vi "DialogCloneClass.vi"(0 "ClassWriterNative.lvclass":refnum<class "ClassWriterNative.lvclass">, 1 "ClassItemRefIn":refnum<vi>, 5 "error in (no error)":errorcluster) -> (14 "ClassWriterGOOP300.lvclassOut":refnum<class "ClassWriterNative.lvclass">, 15 "ClassItemRefOut":refnum<vi>, 16 "NewClassPath":path, 17 "Cancelled":bool, 19 "error out":errorcluster)   [LabVIEW 2014, in "ClassWriterNative.lvclass"]
uses:
  <resource>/Framework/Providers/Open_GDS/ClassProviders/Provider_LvNativeClass/ClassWriterNative_class/ClassWriterNative.lvclass
  <resource>/Framework/Providers/Open_GDS/SubVIs/GOOP_HelpButton.ctl
  <vilib>/Utility/lvfile.llb/NI_FileType.lvlib
panel:
  out "ProductPicture":picture
  in  "_HelpCloneClass":T1
  in  "_UseClassSuffix":string caption="Class Folder Suffix"
  in  "_NewClassPath":path caption="New Class Folder"
  in  "_NewClassName":string caption="New Class Name"
  out "_DubName":string caption="This class already exists"
  in  "_Cancel":bool
  in  "_CloneClass":bool
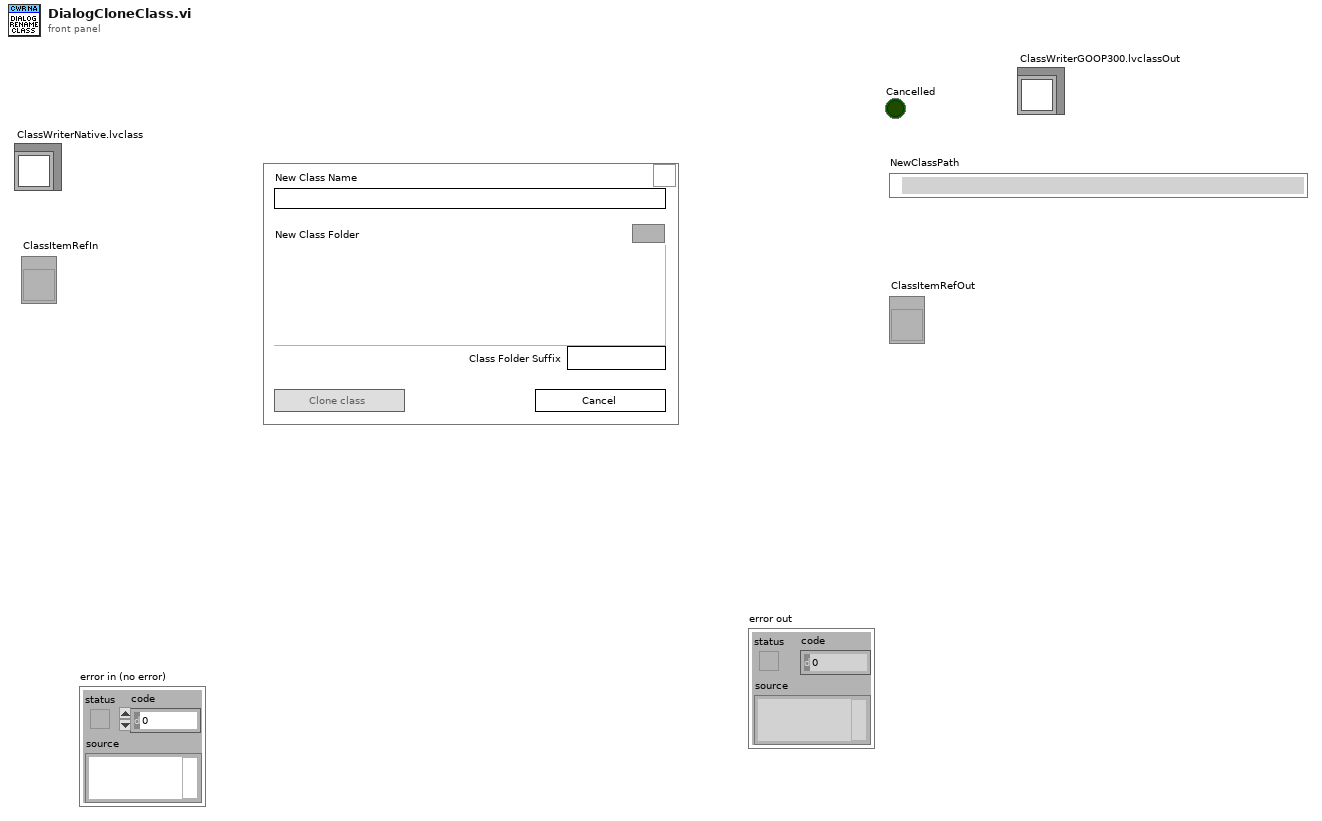
[diagram p1: front panel]
types:
  T1 = typedef "GOOP_HelpButton.ctl" = bool
  T2 = cluster{"Cancel":bool, "OrgClassPath":path, "ClassName":string}
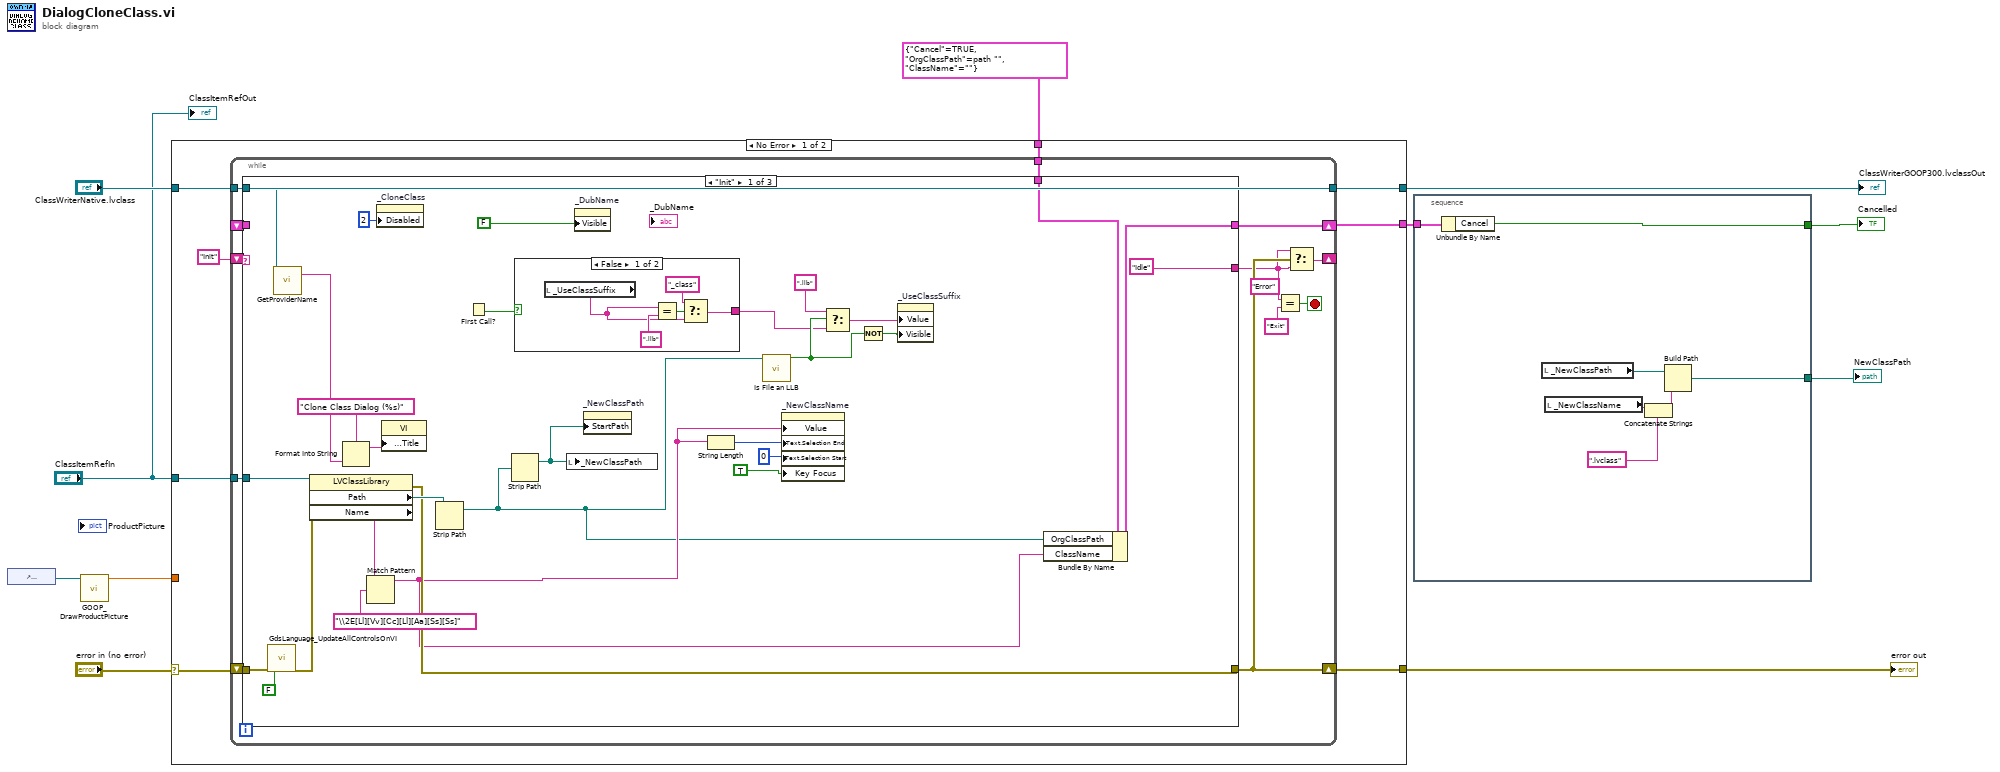
[diagram p0: block diagram]
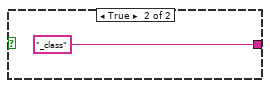
[diagram p2: hidden frame]
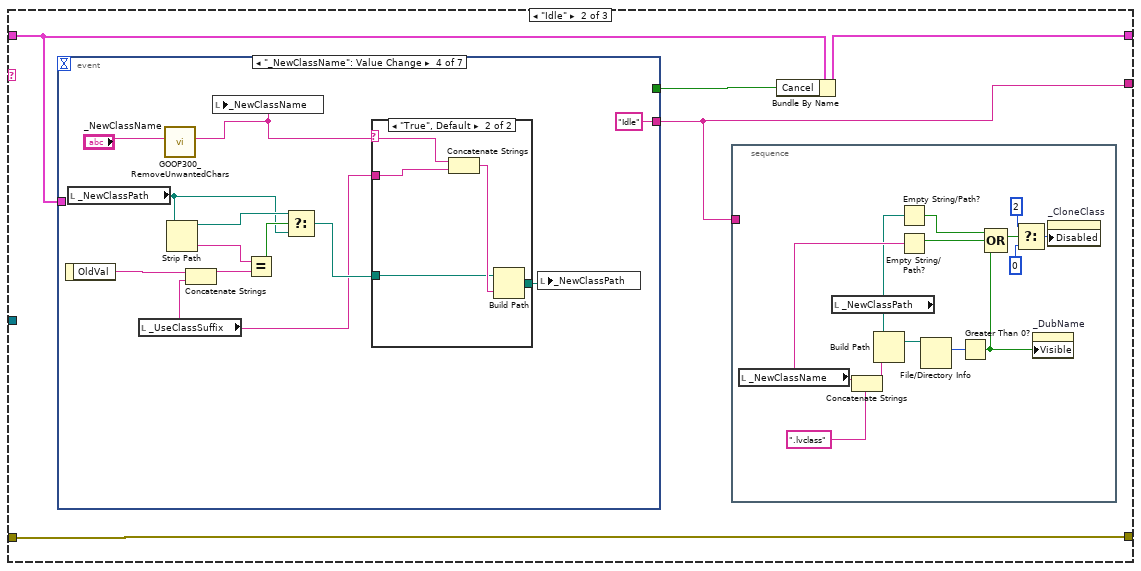
[diagram p3: hidden frame]
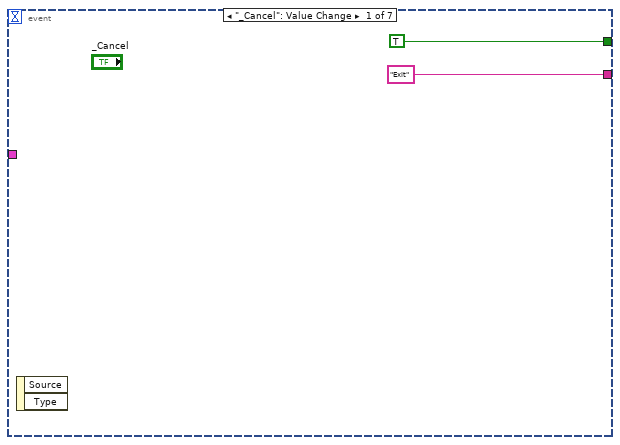
[diagram p4: hidden frame]
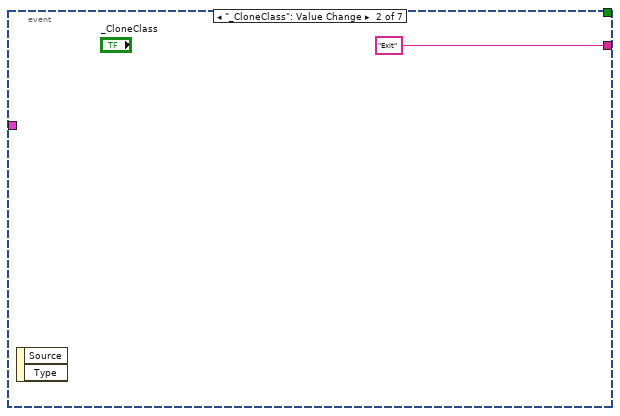
[diagram p5: hidden frame]
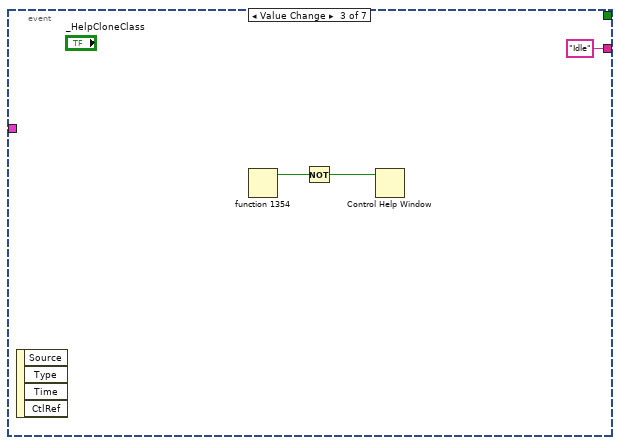
[diagram p6: hidden frame]
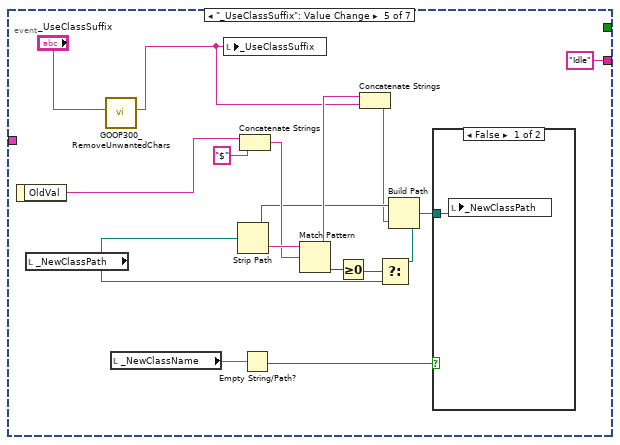
[diagram p8: hidden frame]
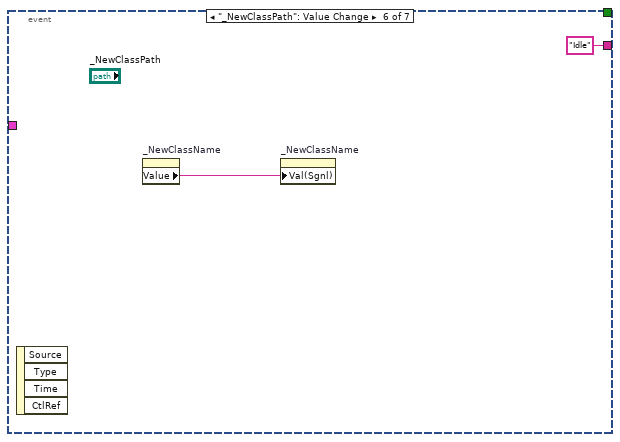
[diagram p10: hidden frame]
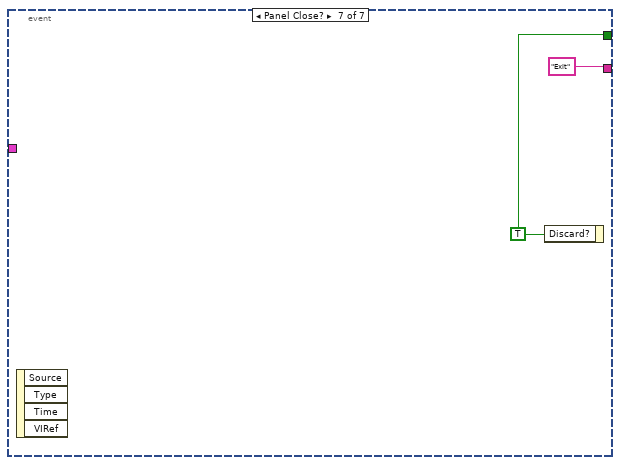
[diagram p11: hidden frame]
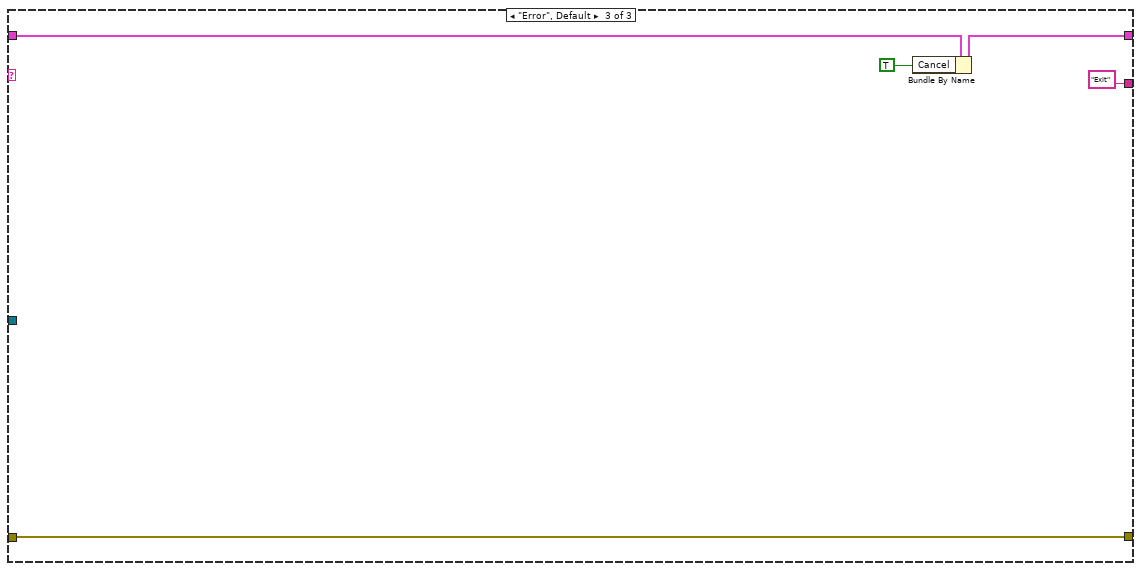
[diagram p12: hidden frame]
diagram:
  n1 = control-ref of="ProductPicture"() -> (w2:refnum<vi>)
  n2 = call <resource>:"GOOP_DrawProductPicture.vi"("ProductPictureControl"=w2) -> ("Zoom Factor"=w1:sgl)  [unwired: 10 in]
  n3 = case shown="No Error" "error in (no error)" {
    selector: "error in (no error)" -> [w19 w137]
    tunnel: "ClassWriterNative.lvclass" -> [w15 w136]
    tunnel: [w18 w137] -> w5
    tunnel: [w16 w136] -> w9
    tunnel: T2 {"Cancel"=TRUE, "OrgClassPath"=path "", "ClassName"=""} ("output cluster") -> [w14 _]
    tunnel: "ClassItemRefIn" -> [w13 _]
    tunnel: [w12 _] -> w8
    tunnel: w1 -> [_ _]
    frame No Error {
      n4 = while {
        shift-right: [w26] -> w18
        shift-left: w19 -> [w32]
        shift-right: [w25] -> _
        shift-left: "Init" -> [w29]
        shift-right: [w30] -> w12
        shift-left: _ -> [w31]
        tunnel: w15 -> [w22]
        tunnel: [w22] -> w16
        tunnel: w14 -> [w21]
        tunnel: w13 -> [w20]
        stop <- w27 stop-if-true
        n5 = case shown="\"Init\"" w29 {
          tunnel: w31 -> [_ w68 w133]
          tunnel: [w60 w70 w132] -> w30
          tunnel: w32 -> [w41 w72 w134]
          tunnel: [w52 w72 w134] -> w26
          tunnel: w22 -> [w43 _ _]
          tunnel: ["Idle" w71 "Exit"] -> w24
          tunnel: w21 -> [w58 _ _]
          tunnel: w20 -> [w59 _ _]
          frame "Init" {
            n6 = call <resource>:"GdsLanguage_UpdateAllControlsOnVI.vi"("error in (no error)"=w41, "CreateLanguageFile(Use this to create a languageFile)"=FALSE) -> ("error out"=w40:errorcluster)  [unwired: 16 in, 1 out]
            n7 = call-dynamic "GetProviderName.vi"("ClassWriterNative in"=w43) -> ("ProviderName"=w42:string)  [unwired: 16 in, 2 out]
            n8 = property class="LVClassLibrary"(reference=w59, error in=w40) -> (error out=w52:errorcluster, "Path"=w56:path, "Name"=w55:string)  [unwired: 1 out]
            n9 = Format Into String(format string="Clone Class Dialog (%s)", w42) -> (resulting string=w45:string)  [unwired: 2 in, 1 out]
            n10 = Match Pattern(string=w55, regular expression="\\2E[Ll][Vv][Cc][Ll][Aa][Ss][Ss]") -> (before substring=w50:string)  [unwired: 1 in, 3 out]
            n11 = property on="_CloneClass" class="Bool"("Disabled"=u8 2) -> ()  [unwired: 2 in, 2 out]
            n12 = property class="VI"("Front Panel.Title"=w45) -> ()  [unwired: 2 in, 2 out]
            n13 = Strip Path(path=w56) -> (stripped path=w33:path)  [unwired: 1 out]
            n14 = First Call?() -> (First Call?: T/F=w48:bool)
            n15 = Strip Path(path=w33) -> (stripped path=w47:path)  [unwired: 1 out]
            n16 = case shown="False" w48 {
              tunnel: [w63 "_class" ("Use Class Prefix")] -> w34
              frame False {
                n17 = local read "_UseClassSuffix"() -> (w62:string)
                n18 = Equal?(x=w62, y=".llb") -> (x = y?=w66:bool)
                n19 = Select(t="_class" ("Use Class Prefix"), s=w66, f=w62) -> (s? t:f=w63:string)
              }
              frame True {
              }
            }
            n20 = local write "_NewClassPath"(w47) -> ()
            n21 = property on="_DubName" class="Str"("Visible"=FALSE) -> ()  [unwired: 2 in, 2 out]
            n22 = property on="_NewClassPath" class="Path"("StartPath"=w47) -> ()  [unwired: 2 in, 2 out]
            n23 = String Length(string=w50) -> (length=w46:i32)
            n24 = call <vilib>:"Is File an LLB.vi"("path"=w33) -> ("Is LLB?"=w35:bool)  [unwired: 9 in, 1 out]
            n25 = property on="_NewClassName" class="Str"("Value"=w50, "Text.Selection End"=w46, "Text.Selection Start"=u32 0 ("Text.Selection:Start"), "Key Focus"=TRUE) -> ()  [unwired: 2 in, 2 out]
            n26 = Select(t=".llb" ("y"), s=w35, f=w34) -> (s? t:f=w36:string)
            n27 = Not(x=w35) -> (.not. x?=w38:bool)
            n28 = property on="_UseClassSuffix" class="Str"("Value"=w36, "Visible"=w38) -> ()  [unwired: 2 in, 2 out]
            n29 = Bundle By Name(cluster=w58, "OrgClassPath"=w33, "ClassName"=w50) -> (w60:T2)
          }
          frame "Idle" {
            n30 = event shown="[3] \"_NewClassName\": Value Change" {
              selector: _ -> [_ _ _ _ _ _ _]
              dyn-events: _ -> [_ _ _ _ _ _ _]
              timeout: _ -> [_ _ _ _ _ _ _]
              tunnel: ["Exit" "Exit" "Idle" "Idle" "Idle" "Idle" "Exit"] -> w71
              tunnel: [TRUE _ _ _ _ _ w130] -> w69
              tunnel: w68 -> [_ _ _ _ _ _ _]
              event "_Cancel": Value Change {
                n31 = event-data() -> ()  [unwired: 1 in, 2 out]
              }
              event "_CloneClass": Value Change {
                n32 = event-data() -> ()  [unwired: 1 in, 2 out]
              }
              event Value Change {
                n33 = event-data() -> ()  [unwired: 1 in, 4 out]
                n34 = fn#1354() -> (1:w91:bool)  [unwired: 1 out]
                n35 = Not(x=w91) -> (.not. x?=w90:bool)
                n36 = Control Help Window(1:w90) -> ()  [unwired: 1 in]
              }
              event "_NewClassName": Value Change {
                n37 = event-data() -> ("OldVal"=w95:string)  [unwired: 1 in]
                n38 = local read "_NewClassPath"() -> (w92:path)
                n39 = local read "_UseClassSuffix"() -> (w94:string)
                n40 = call <resource>:"GOOP300_RemoveUnwantedChars.vi"("StringIn"="_NewClassName") -> ("StringOut"=w96:string)  [unwired: 10 in]
                n41 = Strip Path(path=w92) -> (stripped path=w99:path, name=w101:string)
                n42 = Concatenate Strings(w95, w94) -> (w102:string)
                n43 = local write "_NewClassName"(w96) -> ()
                n44 = Equal?(x=w101, y=w102) -> (x = y?=w100:bool)
                n45 = Select(t=w99, s=w100, f=w92) -> (s? t:f=w98:path)
                n46 = case shown="\"True\", Default" w96 {
                  selector: w96 -> [_ w105]
                  tunnel: [w104 w109] -> w93
                  tunnel: w94 -> [_ w108]
                  tunnel: w98 -> [w104 w106]
                  frame "" {
                  }
                  frame "True", Default {
                    n47 = Concatenate Strings(w105, w108) -> (w107:string)
                    n48 = Build Path(base path=w106, name or relative path=w107) -> (appended path=w109:path)
                  }
                }
                n49 = local write "_NewClassPath"(w93) -> ()
              }
              event "_UseClassSuffix": Value Change {
                n50 = event-data() -> ("OldVal"=w112:string)  [unwired: 1 in]
                n51 = local read "_NewClassPath"() -> (w115:path)
                n52 = call <resource>:"GOOP300_RemoveUnwantedChars.vi"("StringIn"="_UseClassSuffix") -> ("StringOut"=w116:string)  [unwired: 10 in]
                n53 = local read "_NewClassName"() -> (w111:string)
                n54 = local write "_UseClassSuffix"(w116) -> ()
                n55 = Strip Path(path=w115) -> (stripped path=w118:path, name=w124:string)
                n56 = Concatenate Strings(w112, "$" ("string")) -> (w122:string)
                n57 = Empty String/Path?(string/path=w111) -> (empty?=w110:bool)
                n58 = Match Pattern(string=w124, regular expression=w122) -> (before substring=w119:string, offset past match=w123:i32)  [unwired: 1 in, 2 out]
                n59 = Greater Or Equal To 0?(x=w123) -> (x >= 0?=w120:bool)
                n60 = Concatenate Strings(w119, w116) -> (w117:string)
                n61 = Build Path(base path=w118, name or relative path=w117) -> (appended path=w114:path)
                n62 = Select(t=w114, s=w120, f=w115) -> ()  [unwired: 1 out]
                n63 = case shown="False" w110 {
                  tunnel: w114 -> [w126 _]
                  frame False {
                    n64 = local write "_NewClassPath"(w126) -> ()
                  }
                  frame True {
                  }
                }
              }
              event "_NewClassPath": Value Change {
                n65 = event-data() -> ()  [unwired: 1 in, 4 out]
                n66 = property on="_NewClassName" class="Str"() -> ("Value"=w127:string)  [unwired: 2 in, 2 out]
                n67 = property on="_NewClassName" class="Str"("Val(Sgnl)"=w127) -> ()  [unwired: 2 in, 2 out]
              }
              event Panel Close? {
                w130 = TRUE ("Discard?")
                n68 = event-data() -> ()  [unwired: 1 in, 4 out]
                n69 = event-data("Discard?"=w130) -> ()  [unwired: 1 in, 1 out]
              }
            }
            n70 = stacked-sequence {
              tunnel: w71 -> [_]
              frame #0 {
                n71 = local read "_NewClassName"() -> (w76:string)
                n72 = local read "_NewClassPath"() -> (w74:path)
                n73 = Concatenate Strings(w76, ".lvclass" ("string")) -> (w80:string)
                n74 = Build Path(base path=w74, name or relative path=w80) -> (appended path=w79:path)
                n75 = Empty String/Path?(string/path=w74) -> (empty?=w73:bool)
                n76 = Empty String/Path?(string/path=w76) -> (empty?=w75:bool)
                n77 = File/Directory Info(path=w79) -> (size=w78:i64)  [unwired: 1 in, 6 out]
                n78 = Greater Than 0?(x=w78) -> (x > 0?=w77:bool)
                n79 = Compound Arithmetic op=OR(w73, w75, w77) -> (w82:bool)
                n80 = Select(t=u8 2, s=w82, f=u8 0 ("Disabled")) -> (s? t:f=w85:u8)
                n81 = property on="_DubName" class="Str"("Visible"=w77) -> ()  [unwired: 2 in, 2 out]
                n82 = property on="_CloneClass" class="Bool"("Disabled"=w85) -> ()  [unwired: 2 in, 2 out]
              }
            }
            n83 = Bundle By Name(cluster=w68, "Cancel"=w69) -> (w70:T2)
          }
          frame "Error", Default {
            n84 = Bundle By Name(cluster=w133, "Cancel"=TRUE) -> (w132:T2)
          }
        }
        n85 = Equal?(x=w24, y="Exit") -> (x = y?=w27:bool)
        n86 = Select(t="Error", s=w26, f=w24) -> (s? t:f=w25:string)
      }
    }
    frame Error {
    }
  }
  "ClassWriterGOOP300.lvclassOut" <- w9
  "error out" <- w5
  n87 = stacked-sequence {
    tunnel: w8 -> [w143]
    tunnel: [w144] -> w7
    tunnel: [w138] -> w3
    frame #0 {
      n88 = Unbundle By Name(w143) -> ("Cancel"=w144:bool)
      n89 = local read "_NewClassPath"() -> (w142:path)
      n90 = local read "_NewClassName"() -> (w141:string)
      n91 = Concatenate Strings(w141, ".lvclass" ("string")) -> (w140:string)
      n92 = Build Path(base path=w142, name or relative path=w140) -> (appended path=w138:path)
    }
  }
  "Cancelled" <- w7
  "NewClassPath" <- w3
  "ClassItemRefOut" <- "ClassItemRefIn"
